vi "Initialize.vi"(8 "error in (no error)":errorcluster, 11 "Socket in":refnum<class "Socket.lvclass">) -> (0 "error out":errorcluster, 3 "Socket out":refnum<class "Socket.lvclass">)   [LabVIEW 2018, in "Socket.lvclass"]
uses:
  Socket.lvclass
  Socket.lvclass/Socket.ctl
  State Machine/CM_State Machine.lvclass
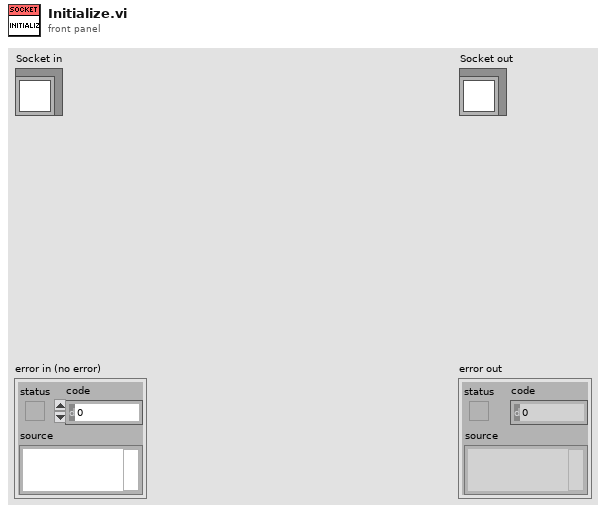
[diagram p1: front panel]
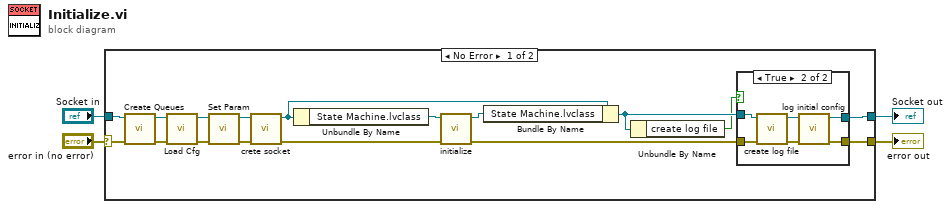
[diagram p0: block diagram]
diagram:
  n1 = case shown="No Error" "error in (no error)" {
    selector: "error in (no error)" -> [w12 w31]
    tunnel: [w14 w31] -> w3
    tunnel: [w15 w30] -> w1
    tunnel: "Socket in" -> [w13 w30]
    frame No Error {
      n2 = call-dynamic "Create Queues.vi"("error in (no error)"=w12, "Socket in"=w13) -> ("error out"=w16:errorcluster, "Socket out"=w17:refnum<class "Socket.lvclass">)  [unwired: 8 in]
      n3 = call-dynamic "Load Cfg.vi"("error in (no error)"=w16, "Socket in"=w17) -> ("error out"=w19:errorcluster, "Socket out"=w21:refnum<class "Socket.lvclass">)  [unwired: 8 in]
      n4 = call-dynamic "Set Param.vi"("error in (no error)"=w19, "Socket in"=w21) -> ("error out"=w18:errorcluster, "Socket out"=w20:refnum<class "Socket.lvclass">)  [unwired: 8 in]
      n5 = call "crete socket.vi"("error in (no error)"=w18, "Socket in"=w20) -> ("error out"=w5:errorcluster, "Socket out"=w9:refnum<class "Socket.lvclass">)  [unwired: 8 in]
      n6 = Unbundle By Name(w9) -> ("State Machine.lvclass"=w8:refnum<class "CM_State Machine.lvclass">)
      n7 = call "initialize.vi"("error in (no error)"=w5, "CM_State Machine in"=w8) -> ("error out"=w6:errorcluster, "CM_State Machine out"=w7:refnum<class "CM_State Machine.lvclass">)  [unwired: 8 in]
      n8 = Bundle By Name(cluster=w9, "State Machine.lvclass"=w7) -> (w11:refnum<class "Socket.lvclass">)
      n9 = Unbundle By Name(w11) -> ("create log file"=w10:bool)
      n10 = case shown="True" w10 {
        tunnel: [w22 w29] -> w15
        tunnel: [w23 w28] -> w14
        tunnel: w6 -> [w23 w24]
        tunnel: w11 -> [w22 w25]
        frame False {
        }
        frame True {
          n11 = call "create log file.vi"("error in (no error)"=w24, "Socket in"=w25) -> ("error out"=w26:errorcluster, "Socket out"=w27:refnum<class "Socket.lvclass">)  [unwired: 8 in]
          n12 = call "log initial config.vi"("error in (no error)"=w26, "Socket in"=w27) -> ("error out"=w28:errorcluster, "Socket out"=w29:refnum<class "Socket.lvclass">)  [unwired: 8 in]
        }
      }
    }
    frame Error {
    }
  }
  "error out" <- w3
  "Socket out" <- w1
